vi "Configure Display.vi"(0 "VISA resource name":refnum<visa-resource-name>, 5 "Display Field (1)":dbl=1.0, 7 "Item (0:Off)":u16(ring) items=["Off", "Input A", "Input B", "Setpoint", "Heater Output"], 9 "Source (1:Kelvin)":u16(ring)=1 items=["Kelvin"=1, "Celsius"=2, "Sensor Units"=3], 11 "error in (no error)":errorcluster) -> (4 "VISA resource name out":refnum<visa-resource-name>, 15 "error out":errorcluster)   [LabVIEW 2019, in "Lake Shore 325.lvlib"]
doc: "This VI configures the Model 325 front panel display settings. In the normal display, the display is divided into four user-configurable fields that can provide temperature readings, setpoint display, and heater status."
uses:
  Lake Shore 325.lvlib
  Instance           1 25Saved   Configure Display .vi
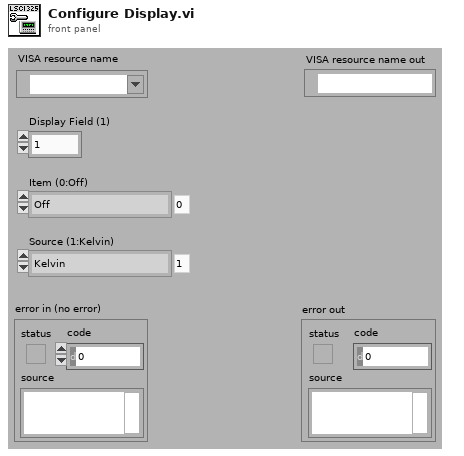
[diagram p1: front panel]
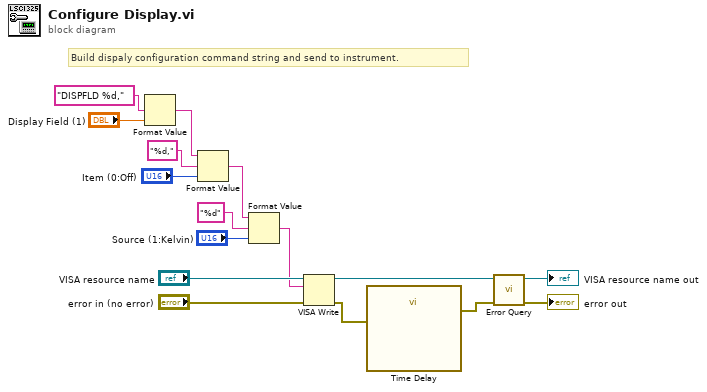
[diagram p0: block diagram]
diagram:
  # "Build dispaly configuration command string and send to instrument."
  n1 = Format Value(format string="DISPFLD %d,", value (0)="Display Field (1)") -> (output string=w7:string)  [unwired: 1 in]
  n2 = Format Value(string ("")=w7, format string="%d,", value (0)="Item (0:Off)") -> (output string=w5:string)
  n3 = Format Value(string ("")=w5, format string="%d", value (0)="Source (1:Kelvin)") -> (output string=w3:string)
  n4 = VISA Write(VISA resource name="VISA resource name", write buffer=w3, error in (no error)="error in (no error)") -> (VISA resource name out=w13:refnum<visa-resource-name>, error out=w2:errorcluster)  [unwired: 1 out]
  n5 = call "Time Delay"("error in (no error)"=w2) -> ("error out"=w1:errorcluster)  [unwired: 10 in]
  n6 = call "Error Query.vi"("error in (no error)"=w1, "VISA resource name"=w13) -> ("error out"=→"error out":errorcluster, "VISA resource name out"=→"VISA resource name out":refnum<visa-resource-name>)  [unwired: 7 in, 1 out]
